vi "Database_Main.vi"(7 "Action":T2, 8 "error in (no error)":errorcluster, 11 "NewFileData":T1) -> (0 "error out":errorcluster, 3 "DataFromFile":T1)   [LabVIEW 2017]
doc: "This is Database module. This module is different from the other modules because it is Functional Global Variable. There was no need to design Database as a separate thread.\n\nBecause it is functional global variable, so it is different thatn the other module, it's icon is gray."
uses:
  Private controls/#TD_Database_DataFromFile_Cluster.ctl
  Private controls/#TD_Database_InnerData.ctl
  <vilib>/Utility/config.llb/NI_LVConfig.lvlib
  <vilib>/Utility/config.llb/Write Key (Boolean).vi
  <vilib>/Utility/config.llb/Read Key (String).vi
  Private controls/#TD_Database_ModuleStates_Enum.ctl
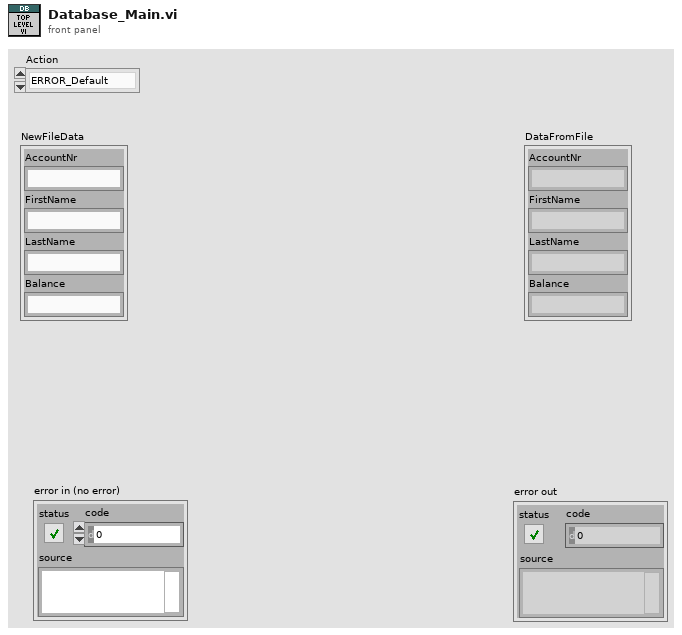
[diagram p1: front panel]
types:
  T1 = typedef "#TD_Database_DataFromFile_Cluster.ctl" = cluster{"AccountNr":string, "FirstName":string, "LastName":string, "Balance":string}
  T2 = typedef "#TD_Database_ModuleStates_Enum.ctl" = enum16{"ERROR_Default", "InitValues", "ReadFile", "GetData", "UpdateFile"}
  T3 = typedef "#TD_Database_InnerData.ctl" = cluster{"Sth":bool, "DataFromFile":T1}
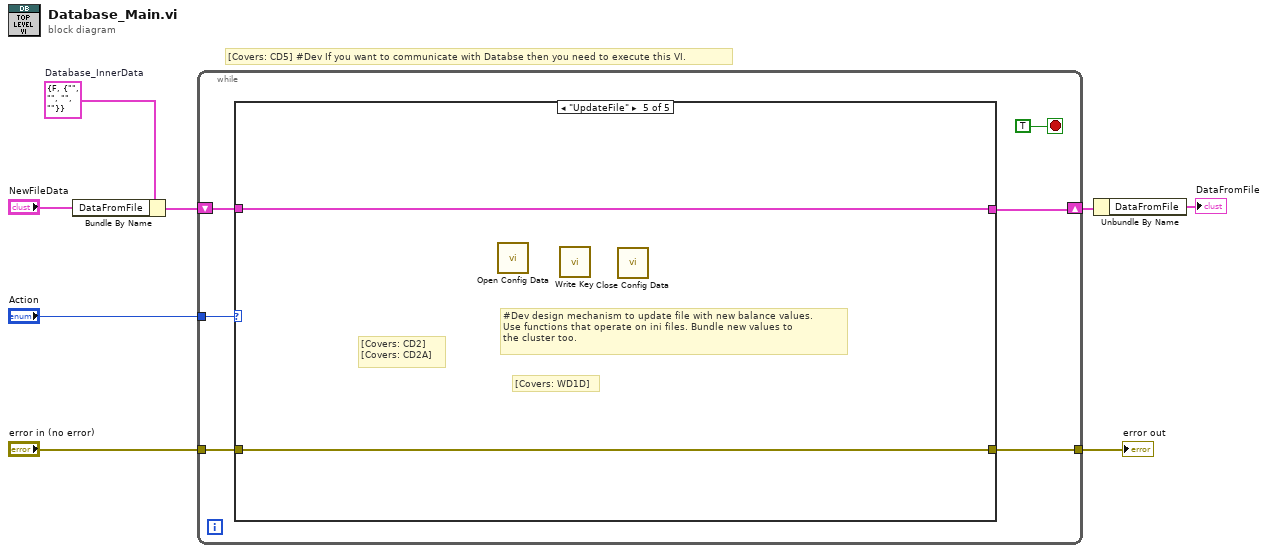
[diagram p0: block diagram]
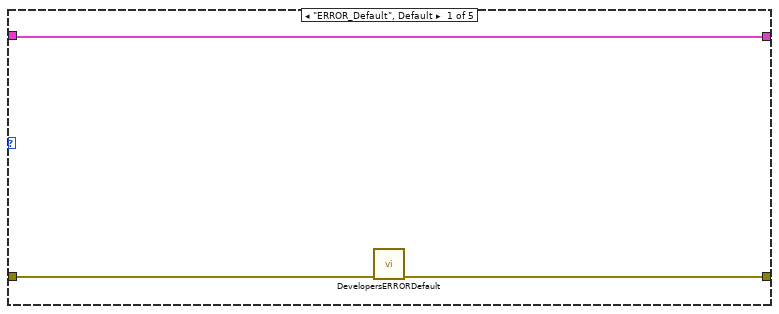
[diagram p2: hidden frame]
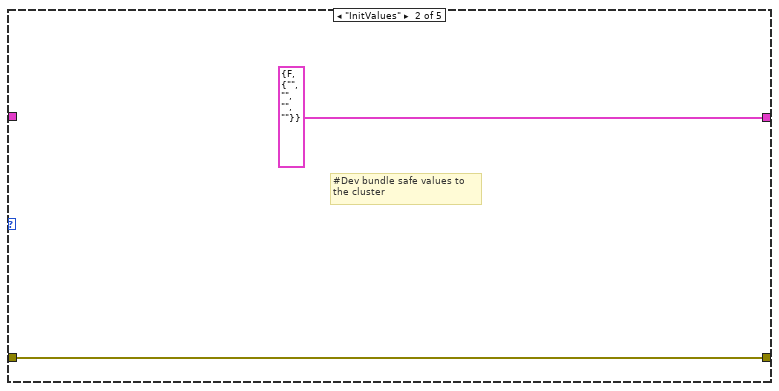
[diagram p3: hidden frame]
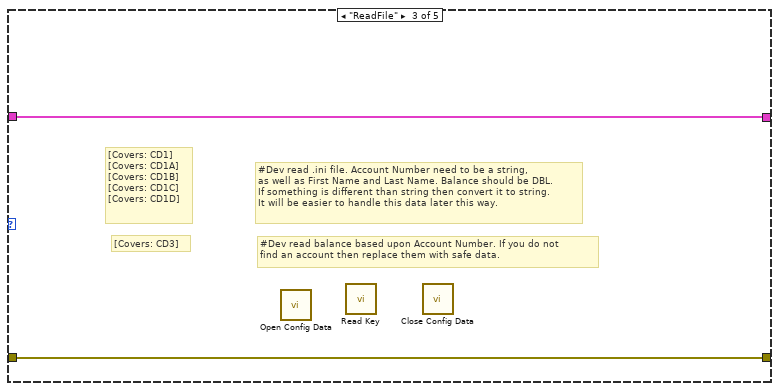
[diagram p4: hidden frame]
diagram:
  w3 = T3 {"Sth"=FALSE, "DataFromFile"={"AccountNr"="", "FirstName"="", "LastName"="", "Balance"=""}}  # Database_InnerData
  # "[Covers: CD5] #Dev If you want to communicate with Databse then you need to execute this VI."
  n1 = Bundle By Name(cluster=w3, "DataFromFile"="NewFileData") -> (w2:T3)
  n2 = while {
    tunnel: "error in (no error)" -> [w13]
    tunnel: [w12] -> w7
    tunnel: "Action" -> [w11]
    shift-right: [w10] -> w5
    shift-left: w2 -> [w9]
    stop <- TRUE stop-if-true
    n3 = case shown="\"UpdateFile\"" w11 {
      tunnel: [w16 w19 w21 w22 w24] -> w12
      tunnel: w13 -> [w17 w19 w21 w22 w24]
      tunnel: [w15 T3 {"Sth"=FALSE, "DataFromFile"={"AccountNr"="", "FirstName"="", "LastName"="", "Balance"=""}} ("Database_InnerData") w20 w23 w25] -> w10
      tunnel: w9 -> [w15 _ w20 w23 w25]
      frame "ERROR_Default", Default {
        n4 = call "DevelopersERRORDefault.vi"("error in (no error)"=w17) -> ("error out"=w16:errorcluster)  [unwired: 10 in]
      }
      frame "InitValues" {
        # "#Dev bundle safe values to \nthe cluster"
      }
      frame "ReadFile" {
        # "#Dev read balance based upon Account Number. If you do not \nfind an account then replace them with safe data."
        # "[Covers: CD3]"
        # "#Dev read .ini file. Account Number need to be a string, \nas well as First Name and Last Name. Balance should be DBL. \nIf something is different than string then convert it to string. \nIt will be easier to handle this data later this way."
        # "[Covers: CD1] \n[Covers: CD1A] \n[Covers: CD1B] \n[Covers: CD1C] \n[Covers: CD1D]"
        n5 = call <vilib>:"Open Config Data.vi"() -> ()  [unwired: 9 in, 3 out]
        n6 = call-poly <vilib>:"Read Key.vi"() -> ()  [unwired: 8 in, 4 out]
        n7 = call <vilib>:"Close Config Data.vi"() -> ()  [unwired: 10 in, 2 out]
      }
      frame "GetData" {
      }
      frame "UpdateFile" {
        # "[Covers: WD1D]"
        # "#Dev design mechanism to update file with new balance values. \nUse functions that operate on ini files. Bundle new values to \nthe cluster too."
        # "[Covers: CD2] \n[Covers: CD2A]"
        n8 = call <vilib>:"Open Config Data.vi"() -> ()  [unwired: 9 in, 3 out]
        n9 = call-poly <vilib>:"Write Key.vi"() -> ()  [unwired: 9 in, 3 out]
        n10 = call <vilib>:"Close Config Data.vi"() -> ()  [unwired: 10 in, 2 out]
      }
    }
  }
  "error out" <- w7
  n11 = Unbundle By Name(w5) -> ("DataFromFile"=→"DataFromFile":T1)
